vi "Windows_Sound_Control.vi"() -> ()   [LabVIEW 2013]
uses:
  user32.dll
panel:
  in  "Snd":bool
  in  "Mute":bool
  in  "Minus":bool
  in  "Plus":bool
  # "Control Master Volume"
  # "Launch Windows Sound Utility"
  # "Run SndVol enables you to \nexplicitly see the value of the\nMaster Volume changing."
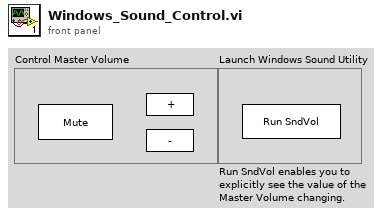
[diagram p1: front panel]
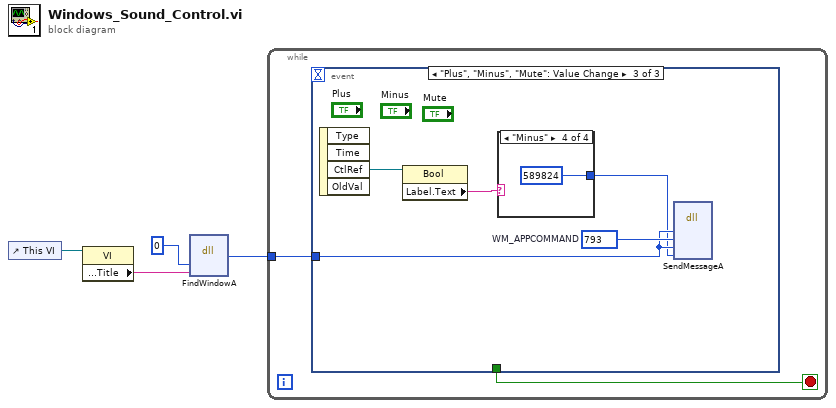
[diagram p0: block diagram]
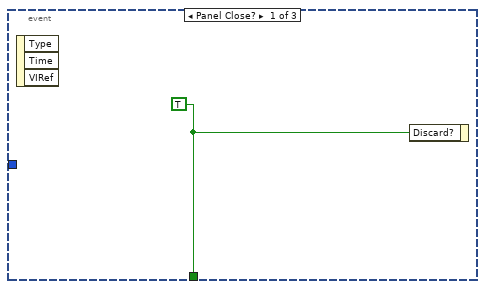
[diagram p2: hidden frame]
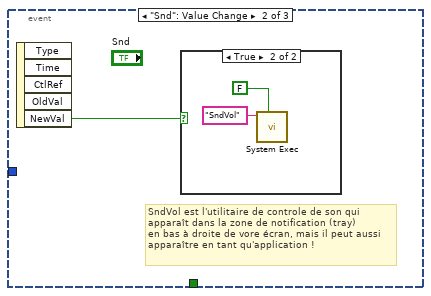
[diagram p3: hidden frame]
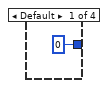
[diagram p5: hidden frame]
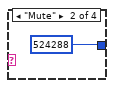
[diagram p6: hidden frame]
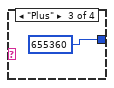
[diagram p7: hidden frame]
diagram:
  n1 = control-ref of="This VI"() -> (w3:refnum<vi>)
  n2 = property class="VI"(reference=w3) -> ("Front Panel.Title"=w2:string)  [unwired: 1 in, 2 out]
  n3 = dll-call lib="user32.dll" fn="FindWindowA" label="FindWindow"("lpszClassName"=0, "lpszWindowName"=w2) -> ("hWnd"=w1:u32)  [unwired: 5 in, 2 out]
  n4 = while {
    tunnel: w1 -> [w5]
    stop <- w6 stop-if-true
    n5 = event shown="[2] \"Plus\", \"Minus\", \"Mute\": Value Change" {
      selector: _ -> [_ _ _]
      dyn-events: _ -> [_ _ _]
      timeout: _ -> [_ _ _]
      tunnel: [w7 _ _] -> w6
      tunnel: w5 -> [_ _ w12]
      event Panel Close? {
        w7 = TRUE
        n6 = event-data() -> ()  [unwired: 1 in, 3 out]
        n7 = event-data("Discard?"=w7) -> ()  [unwired: 1 in, 1 out]
      }
      event "Snd": Value Change {
        # "SndVol est l'utilitaire de controle de son qui\napparaît dans la zone de notification (tray)\nen bas à droite de vore écran, mais il peut aussi\napparaître en tant qu'application !"
        n8 = event-data() -> ("NewVal"=w8:bool)  [unwired: 1 in, 4 out]
        n9 = case shown="True" w8 {
          frame False {
          }
          frame True {
            n10 = call <vilib>:"System Exec.vi"("wait until completion? (T)"=FALSE, "command line"="SndVol") -> ()  [unwired: 6 in, 4 out]
          }
        }
      }
      event "Plus", "Minus", "Mute": Value Change {
        w13 = u32 793  # WM_APPCOMMAND
        n11 = event-data() -> ("CtlRef"=w15:refnum<vi>)  [unwired: 1 in, 3 out]
        n12 = property class="Bool"(reference=w15) -> ("Label.Text"=w14:string)  [unwired: 1 in, 2 out]
        n13 = case shown="\"Minus\"" w14 {
          tunnel: [u32 0 ("APPCOMMAND_VOLUME_DOWN") u32 524288 ("APPCOMMAND_VOLUME_MUTE") u32 655360 ("APPCOMMAND_VOLUME_UP") u32 589824 ("APPCOMMAND_VOLUME_DOWN")] -> w11
          frame Default {
          }
          frame "Mute" {
          }
          frame "Plus" {
          }
          frame "Minus" {
          }
        }
        n14 = dll-call lib="user32.dll" fn="SendMessageA"("hWnd"=w12, "Msg"=w13, "wParam"=w12, "lParam"=w11) -> ()  [unwired: 8 in, 2 out]
      }
    }
  }
